vi "VPA QC Main.vi"() -> ()   [LabVIEW 2013]
uses:
  Controls/VPA QC DAQ Ref Cluster.ctl
  Controls/VPA QC Bool Cluster.ctl
  Controls/VPA QC State Data Cluster.ctl
  Controls/VPA QC General Cluster.ctl
  Controls/VPA QC State Enum.ctl
  Controls/VPA QC DAQ Cmd Enum.ctl
  <vilib>/Utility/miscctls.llb/LVPositionTypeDef.ctl
panel:
  in  "Empty Cluster":T1
  in  "Comments":bool
  out "Version":string
  in  "Print Checklist":bool
  in  "ReqStp":bool
  in  "XDCR PSI 2":dbl
  in  "XDCR PSI 1":dbl
  out "XDCR 2 Scale":dbl=2000.0
  out "XDCR 1 Scale":dbl=2000.0
  out "XDCR 2 Offset":dbl
  out "XDCR 1 Offset":dbl
  in  "FState":dbl
  in  "Exit":bool
  in  "Galil.IGalil":refnum<k7>
  in  "IP Cluster":T5 caption="Select IP to Connect to"
  in  "State Cluster":T1
  out "Bool Cluster":T4
  in  "Galil Ref":refnum<k7>
  in  "VPA Connected?":bool
  in  "IP Address of Pump":string
  in  "DAQ Ref Cluster":T6
  in  "@AN[3]":dbl
  in  "@AN[1]":dbl
  in  "AI1":dbl
  in  "AI0":dbl
  in  "Bin":bool
  in  "Ain":bool
  in  "Bout":bool
  in  "Aout":bool
  in  "_LRB":bool
  in  "_LFB":bool
  in  "_LRA":bool
  in  "_LFA":bool
  in  "MLtot":dbl
  in  "PcurB":dbl
  in  "PcurA":dbl
  in  "Pcur":dbl
  in  "VPA Error":errorcluster
  in  "View/Print Data":bool
  out "VPA":bool
  in  "Final Checklist":bool
  in  "Volume Calibration":bool
  in  "Flow Mode Verification":bool
  in  "Pressure Mode Verification":bool
  in  "Calibrate Pressure Transducers":bool
  in  "Leak Test":bool
  in  "Verify Pump Operation":bool
  in  "Adjust XDCR 0 Offset":bool
  in  "Assembly Checklist":bool
  in  "General Info":bool
  # "VPA Quality Control Checklist"
  # "Assembly Checklist"
  # "Select IP to Connect to:"
  # "Assembly Checklist"
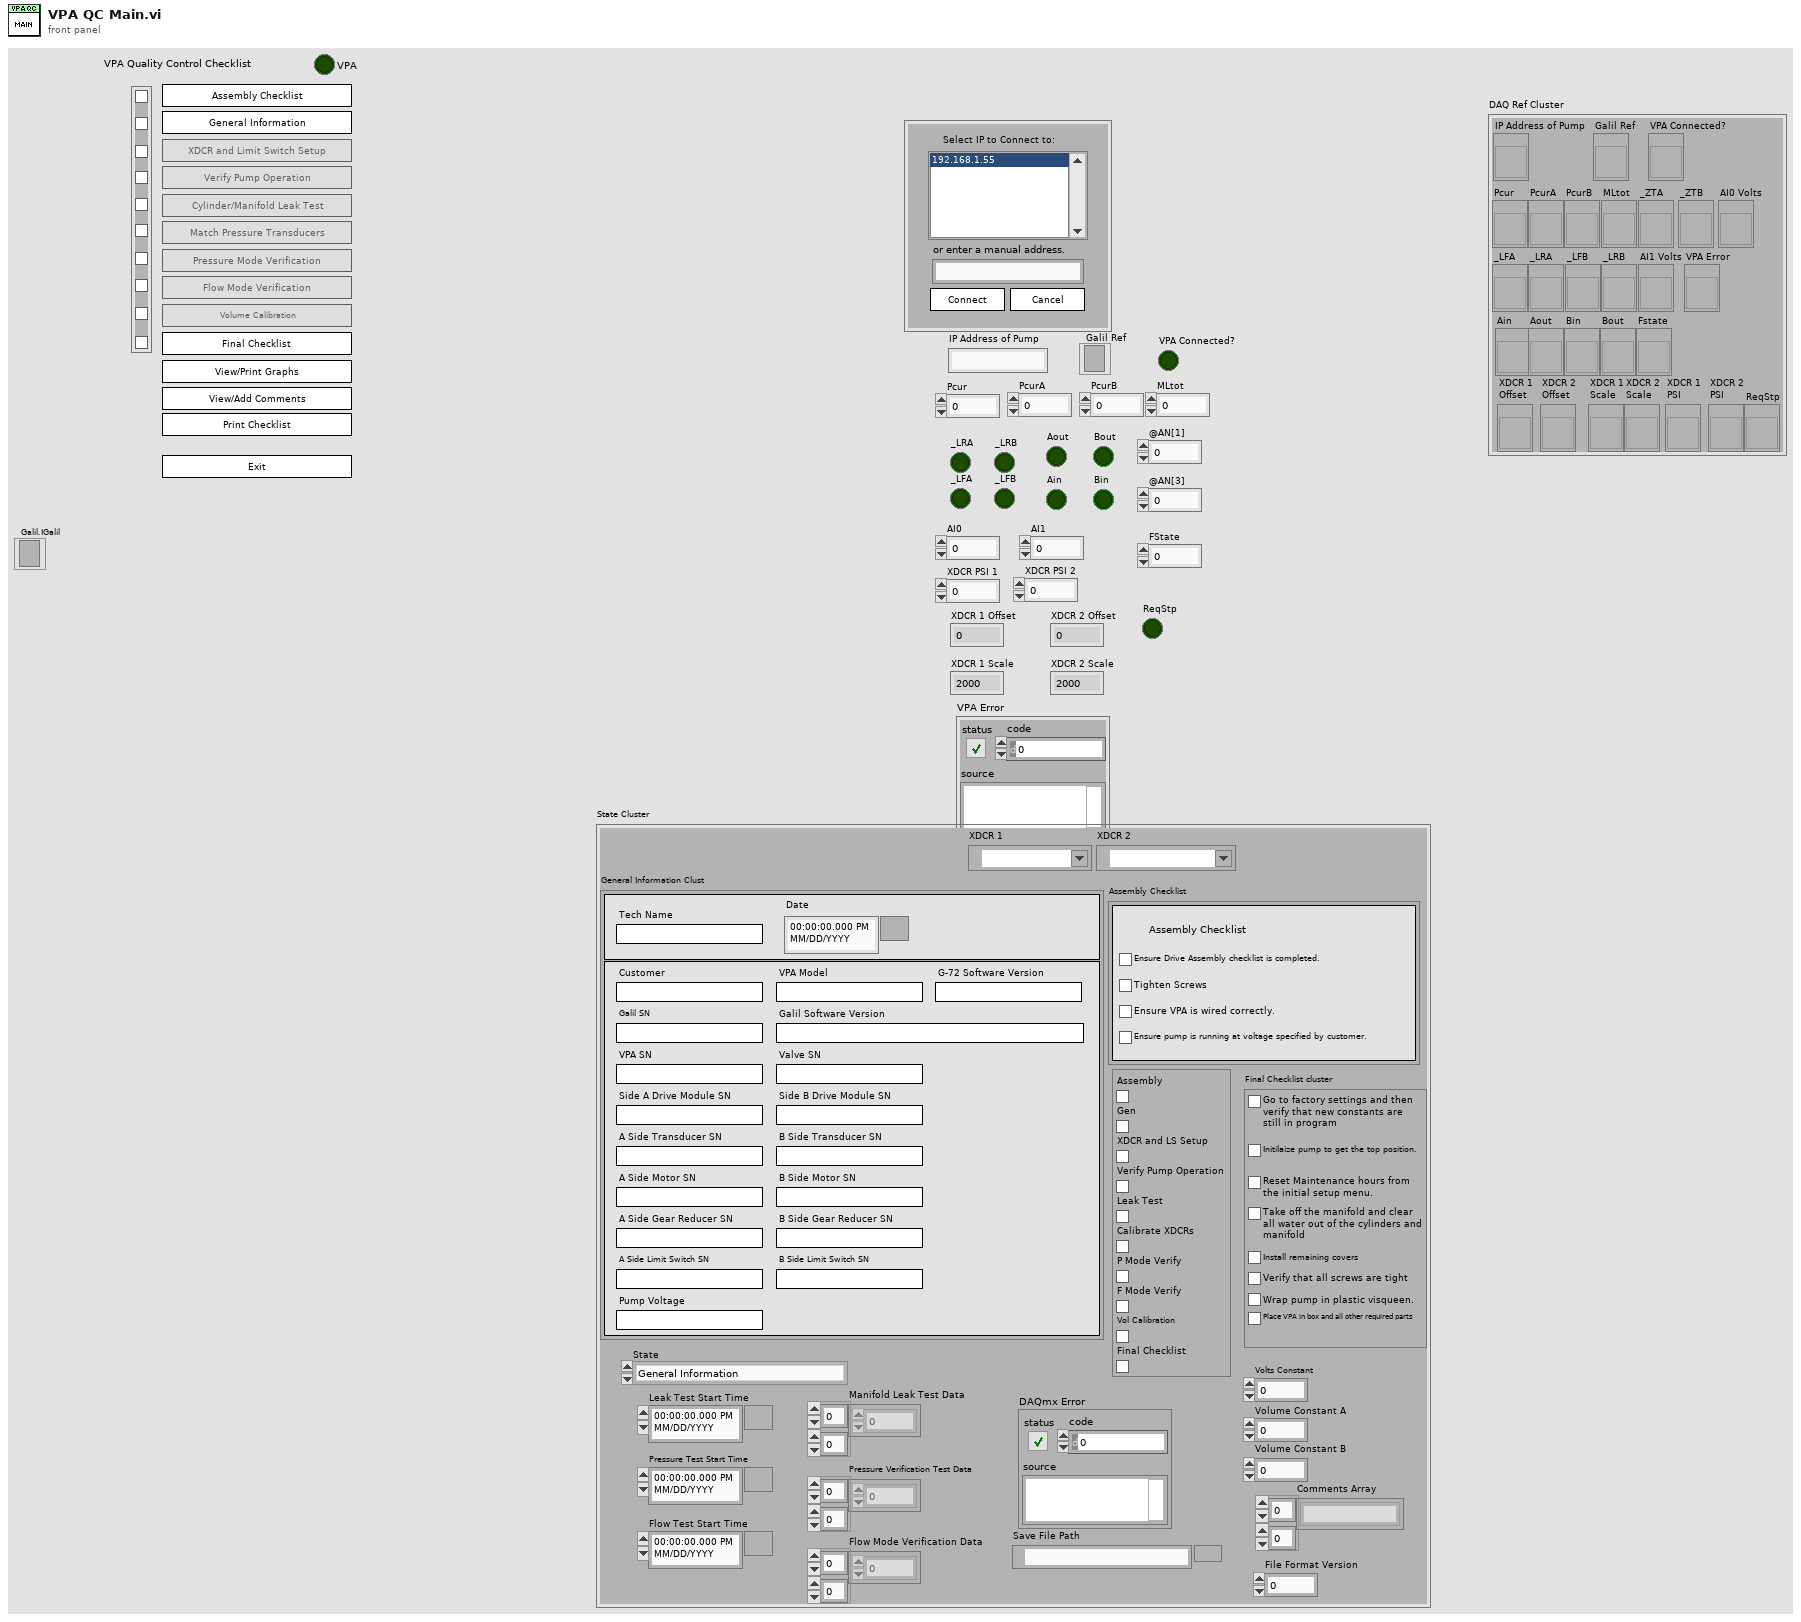
[diagram p1: front panel]
types:
  T1 = typedef "VPA QC State Data Cluster.ctl" = cluster{"XDCR 1":tag, "XDCR 2":tag, "General Information Clust":T2, "Assembly Checklist":cluster{"Ensure Drive Assembly checklist is completed.":bool, "Tighten Screws":bool, "Ensure VPA is wired correctly.":bool, "Ensure pump is running at voltage specified by customer.":bool}, "State":T3, "Manifold Leak Test Data":dbl[][], "Pressure Verification Test Data":dbl[][], "Flow Mode Verification Data":dbl[][], "DAQmx Error":errorcluster, "Bool Cluster":T4, "Leak Test Start Time":timestamp, "Pressure Test Start Time":timestamp, "Flow Test Start Time":timestamp, "Final Checklist cluster":cluster{"Check Fact Rest":bool, "Initialize Pump":bool, "Maintenance Hours":bool, "Clean Water Out":bool, "Covers":bool, "Screws":bool, "Wrap":bool, "Box":bool}, "Volts Constant":dbl, "Volume Constant A":dbl, "Volume Constant B":dbl, "Save File Path":path, "Comments Array":string[][], "File Format Version":u16}
  T2 = typedef "VPA QC General Cluster.ctl" = cluster{"Tech Name":string, "Date":timestamp, "Customer":string, "VPA Model":string, "G-72 Software Version":string, "Galil SN":string, "Galil Software Version":string, "VPA SN":string, "Valve SN":string, "Side A Drive Module SN":string, "Side B Drive Module SN":string, "A Side Transducer SN":string, "B Side Transducer SN":string, "A Side Motor SN":string, "B Side Motor SN":string, "A Side Gear Reducer SN":string, "B Side Gear Reducer SN":string, "A Side Limit Switch SN":string, "B Side Limit Switch SN":string, "Pump Voltage":string}
  T3 = typedef "VPA QC State Enum.ctl" = enum16{"General Information", "XDCR and LS Check", "Check Pump Function", "Manifold/Cylinder Leak Test", "Exit"}
  T4 = typedef "VPA QC Bool Cluster.ctl" = cluster{"Assembly":bool, "Gen":bool, "XDCR and LS Setup":bool, "Verify Pump Operation":bool, "Leak Test":bool, "Calibrate XDCRs":bool, "P Mode Verify":bool, "F Mode Verify":bool, "Vol Calibration":bool, "Final Checklist":bool}
  T5 = cluster{"Available IPs":i32, "Connect":bool, "Cancel":bool, "IP":string}
  T6 = typedef "VPA QC DAQ Ref Cluster.ctl" = cluster{"IP Address of Pump":refnum<vi>, "Galil Ref":refnum<vi>, "VPA Connected?":refnum<vi>, "Pcur":refnum<vi>, "PcurA":refnum<vi>, "PcurB":refnum<vi>, "MLtot":refnum<vi>, "_LFA":refnum<vi>, "_LRA":refnum<vi>, "_LFB":refnum<vi>, "_LRB":refnum<vi>, "_ZTA":refnum<vi>, "_ZTB":refnum<vi>, "AI0 Volts":refnum<vi>, "AI1 Volts":refnum<vi>, "VPA Error":refnum<vi>, "Ain":refnum<vi>, "Aout":refnum<vi>, "Bin":refnum<vi>, "Bout":refnum<vi>, "Fstate":refnum<vi>, "XDCR 1\nOffset":refnum<vi>, "XDCR 2 \nOffset":refnum<vi>, "XDCR 1\nScale":refnum<vi>, "XDCR 2\nScale":refnum<vi>, "XDCR 1\nPSI":refnum<vi>, "XDCR 2\nPSI":refnum<vi>, "ReqStp":refnum<vi>}
  T7 = typedef "VPA QC DAQ Cmd Enum.ctl" = enum16{"Connect", "Disconnect", "Quit", "Close All Valves", "Burn Calibration", "E-Stop", "Set ZC1", "Set ZC0", "Set ZR", "Open Outlet Valves"}
  T8 = typedef "LVPositionTypeDef.ctl" = cluster{"Left":i32, "Top":i32}
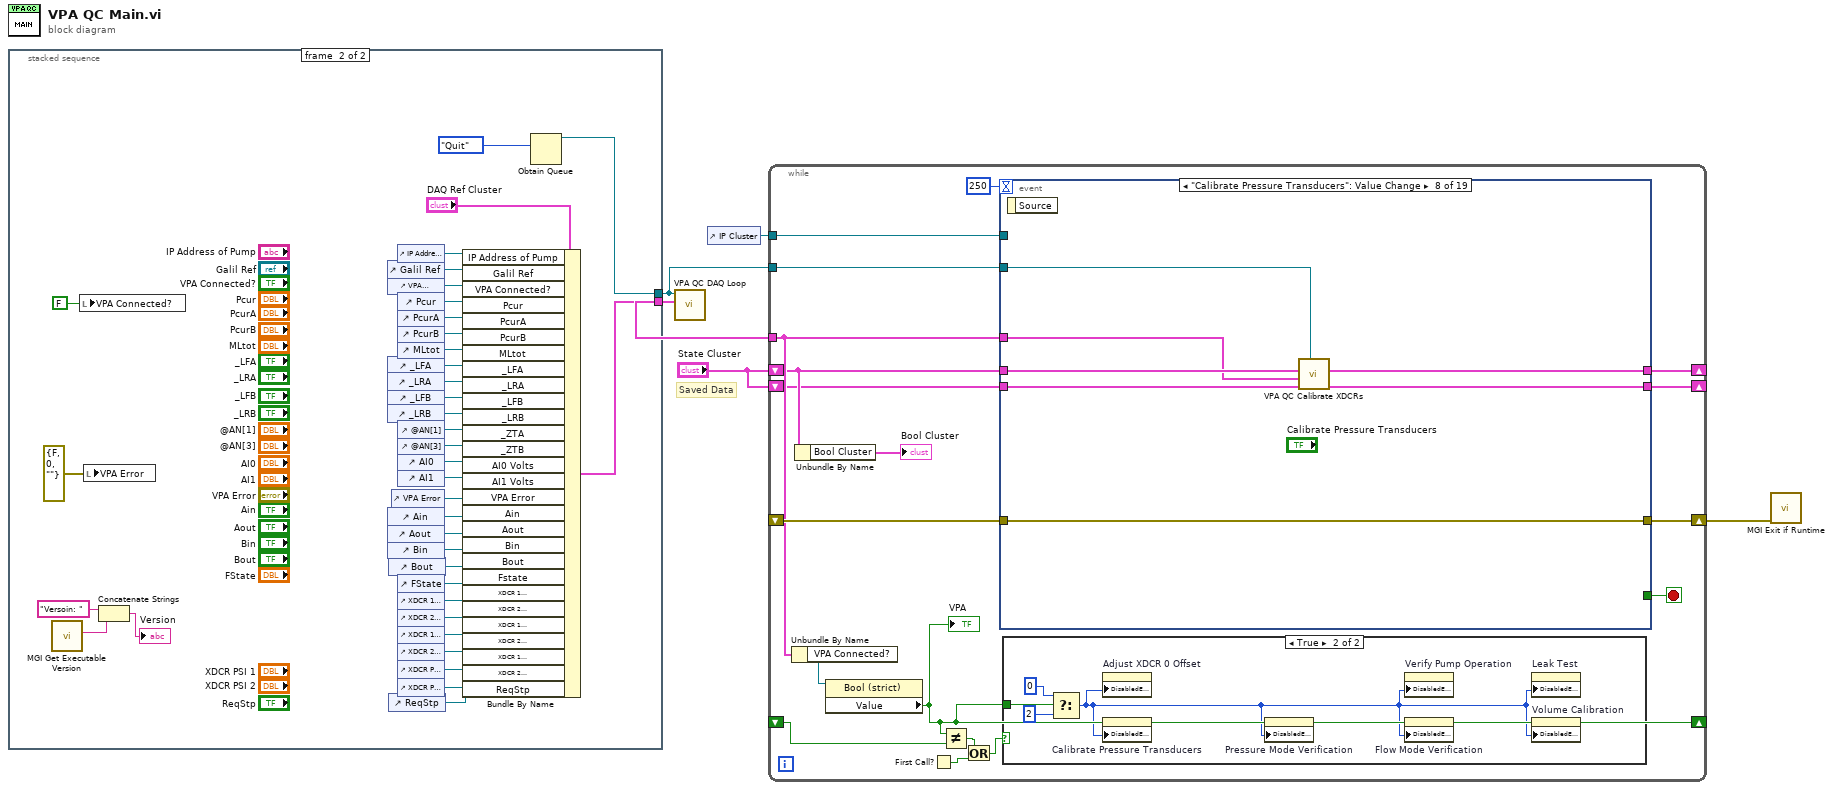
[diagram p0: block diagram]
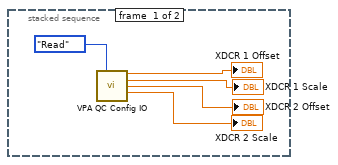
[diagram p2: hidden frame]
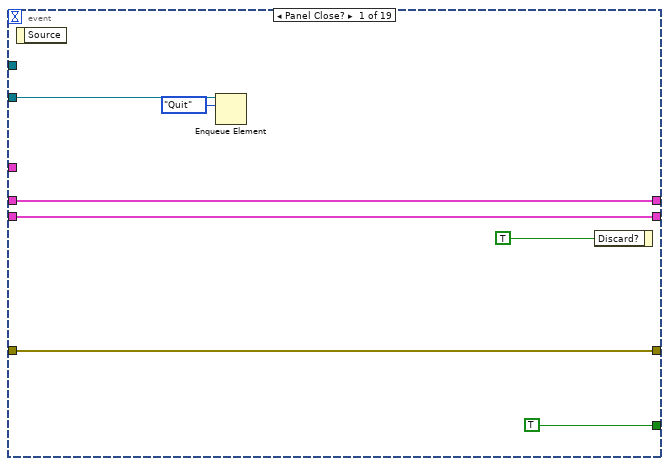
[diagram p4: hidden frame]
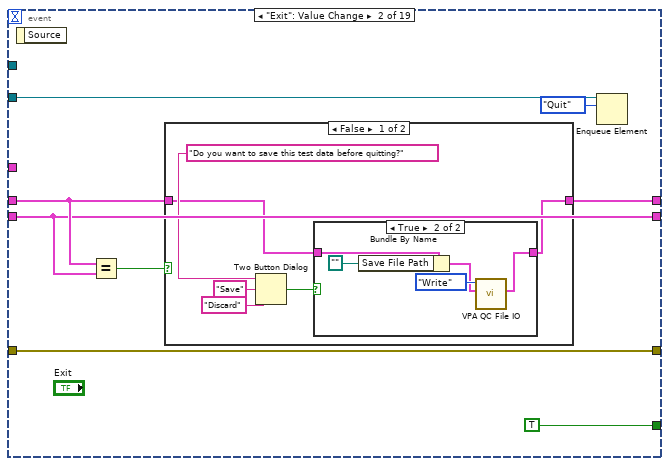
[diagram p5: hidden frame]
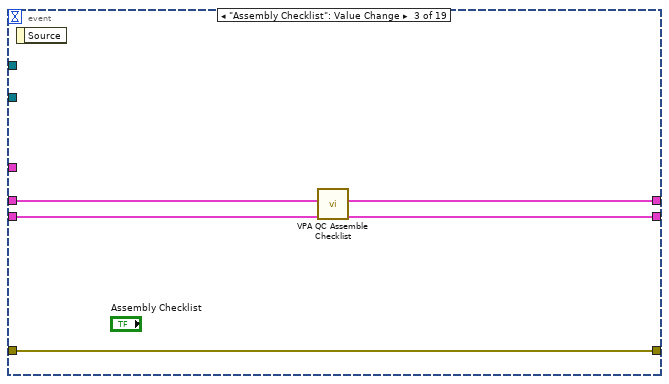
[diagram p8: hidden frame]
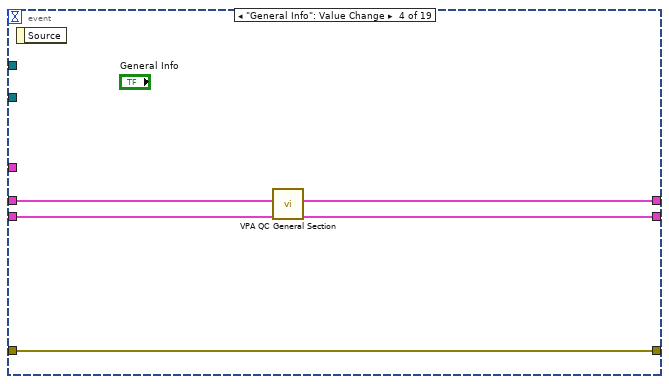
[diagram p9: hidden frame]
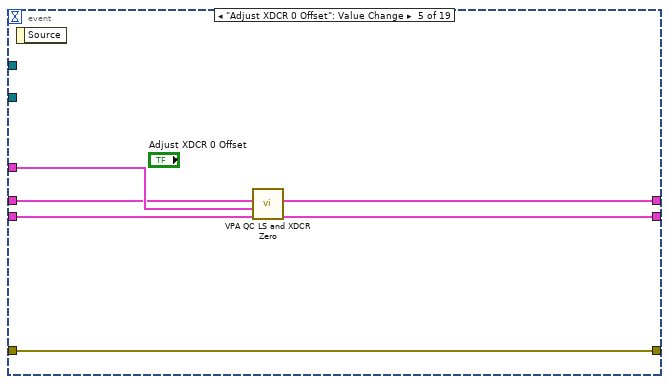
[diagram p10: hidden frame]
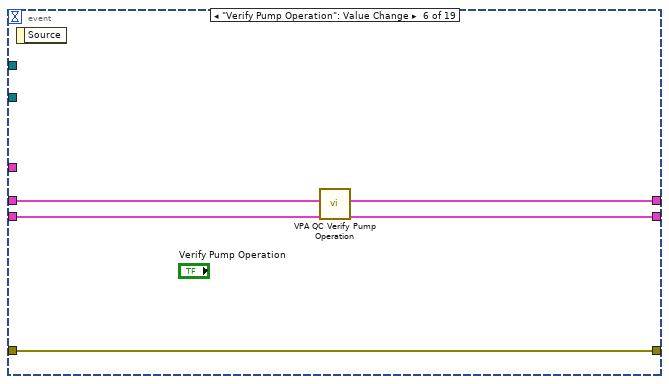
[diagram p11: hidden frame]
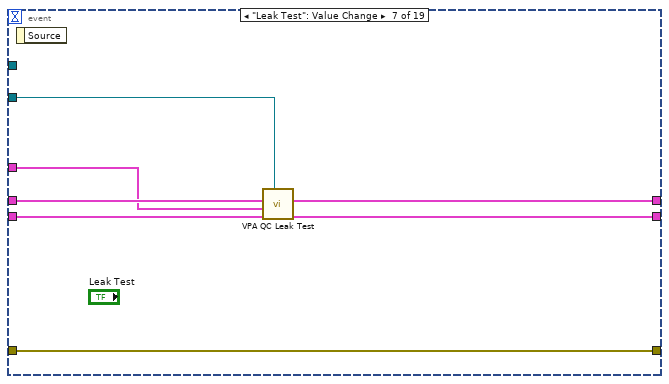
[diagram p12: hidden frame]
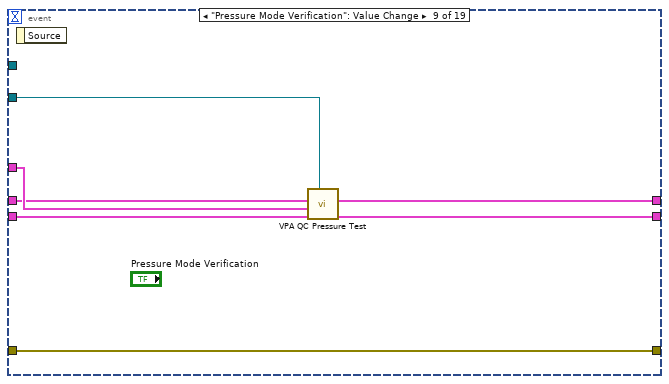
[diagram p13: hidden frame]
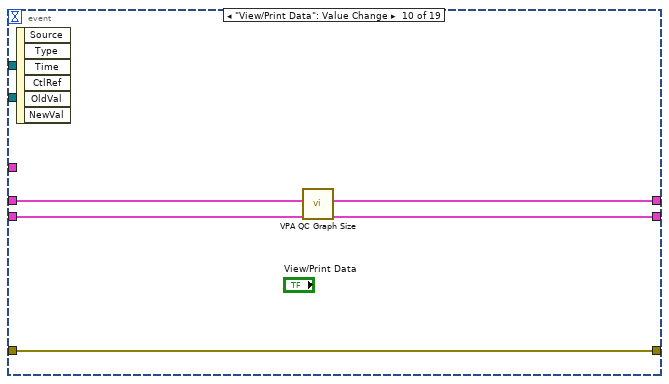
[diagram p14: hidden frame]
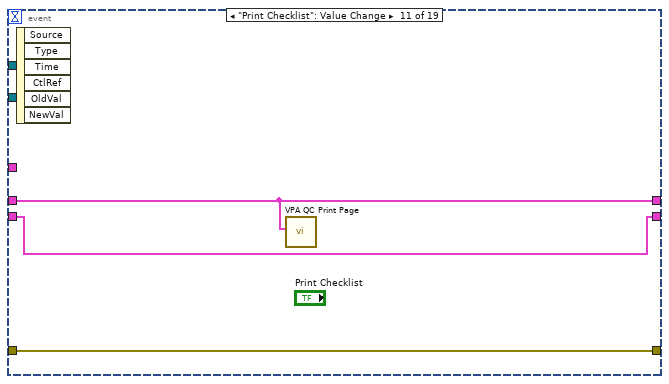
[diagram p15: hidden frame]
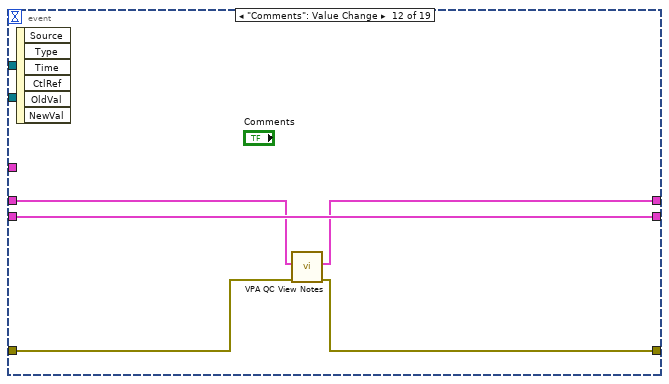
[diagram p16: hidden frame]
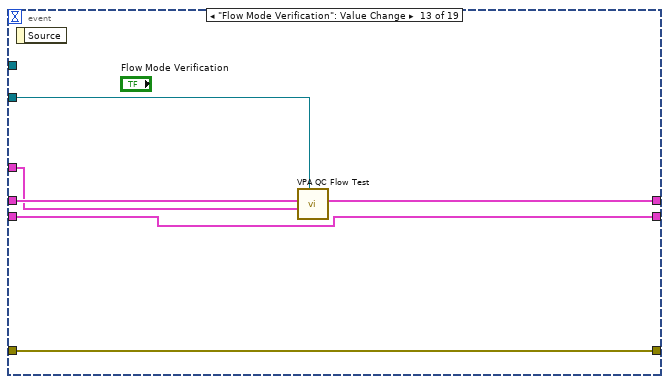
[diagram p17: hidden frame]
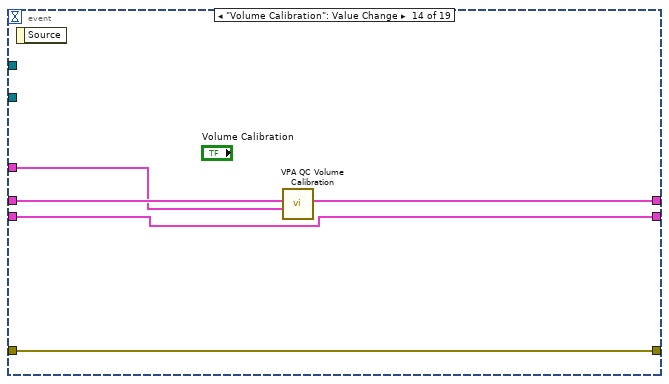
[diagram p18: hidden frame]
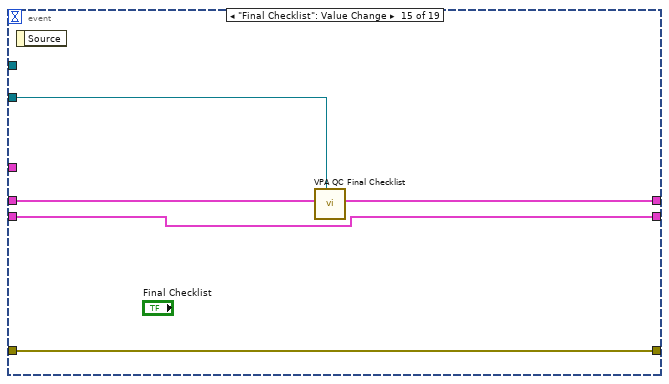
[diagram p19: hidden frame]
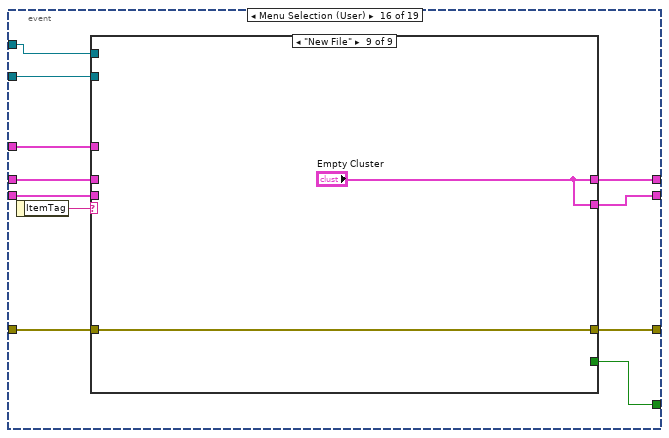
[diagram p20: hidden frame]
diagram:
  # "Saved Data"
  n1 = stacked-sequence {
    tunnel: [_ w26] -> w4
    tunnel: [_ w19] -> w1
    frame #0 {
      n2 = call "VPA QC Config IO.vi"("Function"=enum16{"Read", "Write"}."Read") -> ("XDCR 1 Offset"=→"XDCR 1 Offset":dbl, "XDCR 1 Scale"=→"XDCR 1 Scale":dbl, "XDCR 2 Offset"=→"XDCR 2 Offset":dbl, "XDCR 2 Scale"=→"XDCR 2 Scale":dbl)  [unwired: 11 in]
    }
    frame #1 {
      n3 = call <userlib>:"MGI Get Executable Version.vi"() -> ("Version"=w11:string)  [unwired: 7 in]
      n4 = local write "VPA Connected?"(FALSE ("VPA Connected?")) -> ()
      n5 = local write "VPA Error"(errorcluster {"status"=FALSE, "code"=0, "source"=""} ("VPA Error")) -> ()
      n6 = Concatenate Strings("Versoin: " ("string"), w11) -> (→"Version":string)
      n7 = control-ref of="Galil Ref"() -> (w32:refnum<vi>)
      n8 = control-ref of="VPA Connected?"() -> (w31:refnum<vi>)
      n9 = control-ref of="_LFA"() -> (w42:refnum<vi>)
      n10 = control-ref of="_LRA"() -> (w41:refnum<vi>)
      n11 = control-ref of="_LFB"() -> (w40:refnum<vi>)
      n12 = control-ref of="_LRB"() -> (w39:refnum<vi>)
      n13 = control-ref of="Ain"() -> (w27:refnum<vi>)
      n14 = control-ref of="Aout"() -> (w30:refnum<vi>)
      n15 = control-ref of="Bin"() -> (w29:refnum<vi>)
      n16 = control-ref of="Bout"() -> (w28:refnum<vi>)
      n17 = control-ref of="ReqStp"() -> (w14:refnum<vi>)
      n18 = control-ref of="VPA Error"() -> (w34:refnum<vi>)
      n19 = control-ref of="IP Address of Pump"() -> (w33:refnum<vi>)
      n20 = control-ref of="Pcur"() -> (w46:refnum<vi>)
      n21 = control-ref of="PcurA"() -> (w45:refnum<vi>)
      n22 = control-ref of="PcurB"() -> (w44:refnum<vi>)
      n23 = control-ref of="MLtot"() -> (w43:refnum<vi>)
      n24 = control-ref of="@AN[1]"() -> (w38:refnum<vi>)
      n25 = control-ref of="@AN[3]"() -> (w37:refnum<vi>)
      n26 = control-ref of="AI0"() -> (w36:refnum<vi>)
      n27 = control-ref of="AI1"() -> (w35:refnum<vi>)
      n28 = control-ref of="FState"() -> (w21:refnum<vi>)
      n29 = control-ref of="XDCR 1 Offset"() -> (w25:refnum<vi>)
      n30 = control-ref of="XDCR 2 Offset"() -> (w24:refnum<vi>)
      n31 = control-ref of="XDCR 1 Scale"() -> (w23:refnum<vi>)
      n32 = control-ref of="XDCR 2 Scale"() -> (w22:refnum<vi>)
      n33 = control-ref of="XDCR PSI 1"() -> (w18:refnum<vi>)
      n34 = control-ref of="XDCR PSI 2"() -> (w17:refnum<vi>)
      n35 = Bundle By Name(cluster="DAQ Ref Cluster", "IP Address of Pump"=w33, "Galil Ref"=w32, "VPA Connected?"=w31, "Pcur"=w46, "PcurA"=w45, "PcurB"=w44, "MLtot"=w43, "_LFA"=w42, "_LRA"=w41, "_LFB"=w40, "_LRB"=w39, "_ZTA"=w38, "_ZTB"=w37, "AI0 Volts"=w36, "AI1 Volts"=w35, "VPA Error"=w34, "Ain"=w27, "Aout"=w30, "Bin"=w29, "Bout"=w28, "Fstate"=w21, "XDCR 1\nOffset"=w25, "XDCR 2 \nOffset"=w24, "XDCR 1\nScale"=w23, "XDCR 2\nScale"=w22, "XDCR 1\nPSI"=w18, "XDCR 2\nPSI"=w17, "ReqStp"=w14) -> (w26:T6)
      n36 = Obtain Queue(element data type=VPA_QC_DAQ_Cmd_Enum."Quit" ("element")) -> (queue out=w19:refnum<queue>)  [unwired: 4 in, 2 out]
    }
  }
  n37 = call "VPA QC DAQ Loop.vi"("DAQ Ref Cluster"=w4, "DAQ Q"=w1) -> ()  [unwired: 9 in, 1 out]
  n38 = control-ref of="IP Cluster"() -> (w5:refnum<vi>)
  n39 = while {
    tunnel: w1 -> [w63]
    shift-right: [w64] -> _
    shift-left: "State Cluster" -> [w54]
    tunnel: w5 -> [w62]
    shift-right: [w61] -> w3
    shift-left: _ -> [w60]
    tunnel: w4 -> [w58]
    shift-right: [w55] -> _
    shift-left: _ -> [w56]
    shift-right: [w48] -> _
    shift-left: "State Cluster" -> [w49]
    stop <- w65 stop-if-true
    n40 = Unbundle By Name(w58) -> ("VPA Connected?"=w57:refnum<vi>)
    n41 = Unbundle By Name(w54) -> ("Bool Cluster"=→"Bool Cluster":T4)
    n42 = property class="Bool (strict)"(reference=w57) -> ("Value"=w55:bool)  [unwired: 1 in, 2 out]
    "VPA" <- w55
    n43 = First Call?() -> (First Call?: T/F=w52:bool)
    n44 = Not Equal?(x=w55, y=w56) -> (x != y?=w51:bool)
    n45 = Or(x=w51, y=w52) -> (x .or. y?=w50:bool)
    n46 = event shown="[7] \"Calibrate Pressure Transducers\": Value Change" {
      selector: _ -> [_ _ _ _ _ _ _ _ _ _ _ _ _ _ _ _ _ _ _]
      dyn-events: _ -> [_ _ _ _ _ _ _ _ _ _ _ _ _ _ _ _ _ _ _]
      timeout: 250 -> [_ _ _ _ _ _ _ _ _ _ _ _ _ _ _ _ _ _ _]
      tunnel: [TRUE TRUE _ _ _ _ _ _ _ _ _ _ _ _ _ w170 _ _ _] -> w65
      tunnel: w54 -> [w74 w79 w100 w104 w108 w113 w118 w125 w128 w135 w138 w143 w149 w154 w159 w164 w257 w262 w265]
      tunnel: [w74 w80 w99 w103 w107 w112 w116 w124 w129 w134 w138 w142 w146 w152 w158 w163 w257 w262 w265] -> w64
      tunnel: w63 -> [w73 w83 _ _ _ _ w119 w123 w130 _ _ _ w147 _ w157 w169 w242 _ _]
      tunnel: w62 -> [_ _ _ _ _ _ _ _ _ _ _ _ _ _ _ w168 w256 w259 _]
      tunnel: [w71 w82 w101 w105 w110 w114 w120 w126 w132 w136 w139 w140 w150 w155 w160 w167 w240 w261 w264] -> w61
      tunnel: w60 -> [w71 w82 w101 w105 w110 w114 w120 w126 w132 w136 w139 w141 w150 w155 w160 w166 w246 w261 w264]
      tunnel: w58 -> [_ _ _ _ w109 _ w117 w122 w131 _ _ _ w148 w153 _ w165 w248 _ _]
      tunnel: w49 -> [w70 w78 w98 w102 w106 w111 w115 w121 w127 w133 w137 w144 w145 w151 w156 w162 w232 w258 w263]
      tunnel: [w70 w78 w98 w102 w106 w111 w115 w121 w127 w133 w137 w144 w145 w151 w156 w161 w232 w258 w263] -> w48
      event Panel Close? {
        n47 = event-data() -> ()  [unwired: 1 in, 1 out]
        n48 = Enqueue Element(queue=w73, element=VPA_QC_DAQ_Cmd_Enum."Quit") -> ()  [unwired: 2 in, 3 out]
        n49 = event-data("Discard?"=TRUE) -> ()  [unwired: 1 in, 1 out]
      }
      event "Exit": Value Change {
        n50 = event-data() -> ()  [unwired: 1 in, 1 out]
        n51 = Equal?(x=w79, y=w78) -> (x = y?=w77:bool)
        n52 = case shown="False" w77 {
          tunnel: [w88 w97] -> w80
          tunnel: w79 -> [w87 w97]
          frame False {
            n53 = Two Button Dialog(message="Do you want to save this test data before quitting?", 1:"Discard" ("F button name (\"Cancel\")"), 2:"Save" ("T button name (\"OK\")")) -> (T button?=w89:bool)
            n54 = case shown="True" w89 {
              tunnel: w87 -> [w91 w94]
              tunnel: [w91 w95] -> w88
              frame False {
              }
              frame True {
                n55 = Bundle By Name(cluster=w94, "Save File Path"=path "") -> (w93:T1)
                n56 = call "VPA QC File IO.vi"("State Cluster In"=w93, "Function"=enum16{"Read", "Write"}."Write") -> ("State Cluster Out"=w95:T1)  [unwired: 9 in]
              }
            }
          }
          frame True {
          }
        }
        n57 = Enqueue Element(queue=w83, element=VPA_QC_DAQ_Cmd_Enum."Quit") -> ()  [unwired: 2 in, 3 out]
      }
      event "Assembly Checklist": Value Change {
        n58 = event-data() -> ()  [unwired: 1 in, 1 out]
        n59 = call "VPA QC Assemble Checklist.vi"("State Cluster"=w100) -> ("State Cluster Out"=w99:T1)  [unwired: 10 in]
      }
      event "General Info": Value Change {
        n60 = event-data() -> ()  [unwired: 1 in, 1 out]
        n61 = call "VPA QC General Section.vi"("State Cluster"=w104) -> ("State Cluster Out"=w103:T1)  [unwired: 10 in]
      }
      event "Adjust XDCR 0 Offset": Value Change {
        n62 = event-data() -> ()  [unwired: 1 in, 1 out]
        n63 = call "VPA QC LS and XDCR Zero.vi"("DAQ Ref Cluster"=w109, "State Cluster"=w108) -> ("State Cluster Out"=w107:T1)  [unwired: 9 in]
      }
      event "Verify Pump Operation": Value Change {
        n64 = event-data() -> ()  [unwired: 1 in, 1 out]
        n65 = call "VPA QC Verify Pump Operation.vi"("State Cluster"=w113) -> ("State Cluster Out"=w112:T1)  [unwired: 10 in]
      }
      event "Leak Test": Value Change {
        n66 = event-data() -> ()  [unwired: 1 in, 1 out]
        n67 = call "VPA QC Leak Test.vi"("DAQ Q"=w119, "DAQ Ref Cluster"=w117, "State Cluster"=w118) -> ("State Cluster Out"=w116:T1)  [unwired: 8 in]
      }
      event "Calibrate Pressure Transducers": Value Change {
        n68 = event-data() -> ()  [unwired: 1 in, 1 out]
        n69 = call "VPA QC Calibrate XDCRs.vi"("DAQ Q"=w123, "DAQ Ref Cluster"=w122, "State Cluster"=w125) -> ("State Cluster Out"=w124:T1)  [unwired: 8 in]
      }
      event "Pressure Mode Verification": Value Change {
        n70 = event-data() -> ()  [unwired: 1 in, 1 out]
        n71 = call "VPA QC Pressure Test.vi"("DAQ Q"=w130, "DAQ Ref Cluster"=w131, "State Cluster"=w128) -> ("State Cluster Out"=w129:T1)  [unwired: 8 in]
      }
      event "View/Print Data": Value Change {
        n72 = event-data() -> ()  [unwired: 1 in, 6 out]
        n73 = call "VPA QC Graph Size.vi"("State Cluster"=w135) -> ("State Cluster Out"=w134:T1)  [unwired: 10 in]
      }
      event "Print Checklist": Value Change {
        n74 = event-data() -> ()  [unwired: 1 in, 6 out]
        n75 = call "VPA QC Print Page.vi"("State Cluster"=w138) -> ()  [unwired: 11 in]
      }
      event "Comments": Value Change {
        n76 = event-data() -> ()  [unwired: 1 in, 6 out]
        n77 = call "VPA QC View Notes.vi"("error in (no error)"=w141, "State Cluster in"=w143) -> ("error out"=w140:errorcluster, "State Cluster out"=w142:T1)  [unwired: 8 in]
      }
      event "Flow Mode Verification": Value Change {
        n78 = event-data() -> ()  [unwired: 1 in, 1 out]
        n79 = call "VPA QC Flow Test.vi"("DAQ Q"=w147, "DAQ Ref Cluster"=w148, "State Cluster"=w149) -> ("State Cluster Out"=w146:T1)  [unwired: 8 in]
      }
      event "Volume Calibration": Value Change {
        n80 = event-data() -> ()  [unwired: 1 in, 1 out]
        n81 = call "VPA QC Volume Calibration.vi"("DAQ Ref Cluster"=w153, "State In"=w154) -> ("State Out"=w152:T1)  [unwired: 9 in]
      }
      event "Final Checklist": Value Change {
        n82 = event-data() -> ()  [unwired: 1 in, 1 out]
        n83 = call "VPA QC Final Checklist.vi"("DAQ Q"=w157, "State Cluster"=w159) -> ("State Cluster Out"=w158:T1)  [unwired: 9 in]
      }
      event Menu Selection (User) {
        n84 = event-data() -> ("ItemTag"=w171:string)  [unwired: 1 in]
        n85 = case shown="\"New File\"" w171 {
          tunnel: [TRUE _ _ _ _ _ _ _ _] -> w170
          tunnel: w169 -> [w176 _ w208 _ _ _ _ _ _]
          tunnel: w168 -> [_ w202 _ _ _ _ _ _ _]
          tunnel: [w174 w190 w205 w211 w215 w219 w225 w229 w231] -> w167
          tunnel: w166 -> [w174 _ w206 w211 w215 w219 w225 w229 w231]
          tunnel: w165 -> [_ _ _ _ w214 _ _ _ _]
          tunnel: w164 -> [w173 w179 w204 w210 w213 w217 w221 w228 _]
          tunnel: [w173 w179 w204 w210 w213 w216 w223 w226 "Empty Cluster"] -> w163
          tunnel: w162 -> [w172 w178 w203 w209 w212 _ _ _ _]
          tunnel: [w172 w178 w203 w209 w212 w216 w223 w226 "Empty Cluster"] -> w161
          frame "Exit", Default {
            n86 = Enqueue Element(queue=w176, element=VPA_QC_DAQ_Cmd_Enum."Quit") -> ()  [unwired: 2 in, 3 out]
          }
          frame "Connect" {
            w184 = refnum<vi> refnum  # Boolean
            w198 = refnum<vi> refnum  # ListBox
            n87 = property class="Clust"(reference=w202, "Position"=T8 {"Left"=52, "Top"=76}) -> ("Controls[]"=w200:refnum<vi>[])  [unwired: 1 in, 2 out]
            n88 = Automation Open(Automation Refnum="Galil.IGalil") -> (Automation Refnum=w194:refnum<k7>, error out=w195:errorcluster)  [unwired: 1 in, 2 out]
            n89 = invoke on="Invoke Node" class="IGalil" method="addresses"(reference=w194, error in=w195) -> (reference out=w192:refnum<k7>, error out=w191:errorcluster, "addresses"=w193:variant)  [unwired: 1 in]
            n90 = Index Array(array=w200) -> (element #1=w199:refnum<vi>, element #2=w185:refnum<vi>)  [unwired: 2 in]
            n91 = To More Specific Class(target class=w198, reference=w199) -> (specific class reference=w197:refnum<vi>)  [unwired: 1 in, 1 out]
            n92 = Variant To Data(type=string[] [] ("Item Names"), Variant=w193) -> (data=w180:string[])  [unwired: 1 in, 1 out]
            n93 = Array Size(array=w180) -> (size(s)=w189:i32)
            n94 = property class="LstBox"(reference=w197, "Item Names"=w180) -> ()  [unwired: 1 in, 2 out]
            n95 = Equal To 0?(x=w189) -> (x = 0?=w188:bool)
            n96 = Select(t=2, s=w188, f=0) -> (s? t:f=w182:i32)
            n97 = Close Reference(reference=w192, error in (no error)=w191) -> (error out=w190:errorcluster)
            n98 = To More Specific Class(target class=w184, reference=w185) -> (specific class reference=w183:refnum<vi>)  [unwired: 1 in, 1 out]
            n99 = property class="Bool"(reference=w183, "DisabledEnum"=w182) -> ()  [unwired: 1 in, 2 out]
          }
          frame "Disconnect" {
            n100 = Enqueue Element(queue=w208, element=VPA_QC_DAQ_Cmd_Enum."Disconnect", error in (no error)=w206) -> (error out=w205:errorcluster)  [unwired: 1 in, 2 out]
          }
          frame "View Data" {
          }
          frame "XDCR Setup" {
            n101 = call "VPA QC XDCR Setup.vi"("DAQ Ref Cluster"=w214) -> ()  [unwired: 11 in]
          }
          frame "Save" {
            n102 = call "VPA QC File IO.vi"("State Cluster In"=w217, "Function"=enum16{"Read", "Write"}."Write") -> ("State Cluster Out"=w216:T1)  [unwired: 9 in]
          }
          frame "Save as" {
            n103 = Bundle By Name(cluster=w221, "Save File Path"=path "") -> (w220:T1)
            n104 = call "VPA QC File IO.vi"("State Cluster In"=w220, "Function"=enum16{"Read", "Write"}."Write") -> ("State Cluster Out"=w223:T1)  [unwired: 9 in]
          }
          frame "Load" {
            n105 = call "VPA QC File IO.vi"("State Cluster In"=w228, "Function"=enum16{"Read", "Write"}."Read") -> ("State Cluster Out"=w226:T1)  [unwired: 9 in]
          }
          frame "New File" {
          }
        }
      }
      event "IP Cluster.Available IPs": Double Click; "IP Cluster.Connect": Value Change {
        w254 = refnum<vi> refnum  # ListBox
        # "Check for valid IP format"
        n106 = event-data() -> ()  [unwired: 1 in, 4 out]
        n107 = Unbundle By Name(w248) -> ("IP Address of Pump"=w247:refnum<vi>)
        n108 = property class="Clust"(reference=w256, "Position"=T8 {"Left"=812, "Top"=76}) -> ("Controls[]"=w253:refnum<vi>[])  [unwired: 1 in, 2 out]
        n109 = Unbundle By Name("IP Cluster") -> ("IP"=w234:string)
        n110 = Index Array(array=w253) -> (element=w255:refnum<vi>)  [unwired: 1 in]
        n111 = To More Specific Class(target class=w254, reference=w255, error in=w246) -> (specific class reference=w251:refnum<vi>, error out=w245:errorcluster)
        n112 = Match Pattern(string=w234, regular expression="[0-9]+[.][0-9]+[.][0-9]+[.][0-9]+") -> (offset past match=w237:i32)  [unwired: 1 in, 3 out]
        n113 = property class="LstBox"(reference=w251, error in=w245) -> (error out=w244:errorcluster, "Item Names"=w250:string[], "Active Row"=w249:i32)  [unwired: 1 out]
        n114 = Less Than 0?(x=w237) -> (x < 0?=w236:bool)
        n115 = Index Array(array=w250, index=w249) -> (element=w235:string)
        n116 = Select(t=w235, s=w236, f=w234) -> (s? t:f=w233:string)
        n117 = property class="Str"(reference=w247, error in=w244, "Value"=w233) -> (error out=w243:errorcluster)  [unwired: 1 out]
        n118 = Enqueue Element(queue=w242, element=VPA_QC_DAQ_Cmd_Enum."Connect", error in (no error)=w243) -> (error out=w240:errorcluster)  [unwired: 1 in, 2 out]
      }
      event "IP Cluster.Cancel": Value Change {
        n119 = event-data() -> ()  [unwired: 1 in, 6 out]
        n120 = property class="Clust"(reference=w259, "Position"=T8 {"Left"=812, "Top"=76}) -> ()  [unwired: 1 in, 2 out]
      }
      event Timeout {
        n121 = event-data() -> ()  [unwired: 1 in, 3 out]
      }
    }
    n122 = case shown="True" w50 {
      tunnel: w55 -> [_ w69]
      frame False {
      }
      frame True {
        n123 = Select(t=0, s=w69, f=2) -> (s? t:f=w66:i32)
        n124 = property on="Adjust XDCR 0 Offset" class="Bool"("DisabledEnum"=w66) -> ()  [unwired: 2 in, 2 out]
        n125 = property on="Calibrate Pressure Transducers" class="Bool"("DisabledEnum"=w66) -> ()  [unwired: 2 in, 2 out]
        n126 = property on="Pressure Mode Verification" class="Bool"("DisabledEnum"=w66) -> ()  [unwired: 2 in, 2 out]
        n127 = property on="Verify Pump Operation" class="Bool"("DisabledEnum"=w66) -> ()  [unwired: 2 in, 2 out]
        n128 = property on="Flow Mode Verification" class="Bool"("DisabledEnum"=w66) -> ()  [unwired: 2 in, 2 out]
        n129 = property on="Leak Test" class="Bool"("DisabledEnum"=w66) -> ()  [unwired: 2 in, 2 out]
        n130 = property on="Volume Calibration" class="Bool"("DisabledEnum"=w66) -> ()  [unwired: 2 in, 2 out]
      }
    }
  }
  n131 = call <userlib>:"MGI Exit if Runtime.vi"("Error In (Dependency Only)"=w3) -> ()  [unwired: 11 in]
